vi "Module Top Level.vi"(8 "error in":errorcluster) -> (0 "error out":errorcluster)   [LabVIEW 2018, in "UDP Writer.lvlib"]
doc: "This is the top level VI for this module. It uses a queue for communications and is stopped user a user event. The general architecture is similar to a simple queued message handler.\n\nThe VIs associated with this module are organized in a LabVIEW Library."
uses:
  UDP Writer.lvlib
  Private Controls/Host Comms Data.ctl
  Top Level/Shared Controls/All Data Cluster.ctl
  Top Level/Shared Controls/Acq Data.ctl
  Private Controls/Module Data.ctl
  Private Controls/Module Action.ctl
panel:
  out "Connected?":bool
  # "UDP Writer"
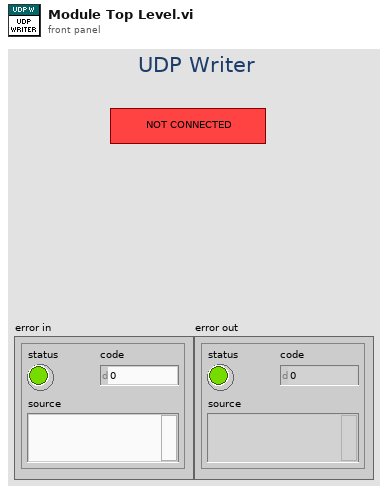
[diagram p1: front panel]
types:
  T1 = typedef "UDP Writer.lvlib/Host Comms Data.ctl" = cluster{"Connected?":bool, "connection ID":refnum<k16>, "PC IP":string, "PC Port":u16, "All Data Cluster":T2}
  T2 = typedef "All Data Cluster.ctl" = cluster{"AI":T3, "Accel Data":cluster{"Accel RMS(in/sec2)":dbl[], "Accel Peak(in/sec2)":dbl[], "Velocity RMS(in/sec)":dbl[], "Velocity Peak(in/sec)":dbl[]}, "Temps":cluster{"01-00-9213":dbl[], "01-01-9213":dbl[], "01-02-9213":dbl[]}, "00-03-9402(RPM)":dbl[], "02-04-9871":dbl[], "ARINC":sgl[]}
  T3 = typedef "Acq Data.ctl" = cluster{"00-00-9220":dbl[], "00-01-9220":dbl[], "02-02-9219":dbl[], "02-03-9227":dbl[], "02-05-9205":dbl[]}
  T4 = cluster{"z0":dbl, "dz":dbl, "plots":cluster{"x0":dbl, "dx":dbl, "Y":dbl[]}[]}
  T5 = cluster{"Accel RMS(in/sec2)":dbl[], "Accel Peak(in/sec2)":dbl[], "Velocity RMS(in/sec)":dbl[], "Velocity Peak(in/sec)":dbl[]}
  T6 = typedef "UDP Writer.lvlib/Module Data.ctl" = cluster{"Data":variant, "Action":T7}
  T7 = typedef "UDP Writer.lvlib/Module Action.ctl" = enum16{"Init", "Update ARINC", "Update Waterfall", "Update RPMs", "Update Temps", "Update Modbus", "Update AI", "Update Vibs", "Write", "Error"}
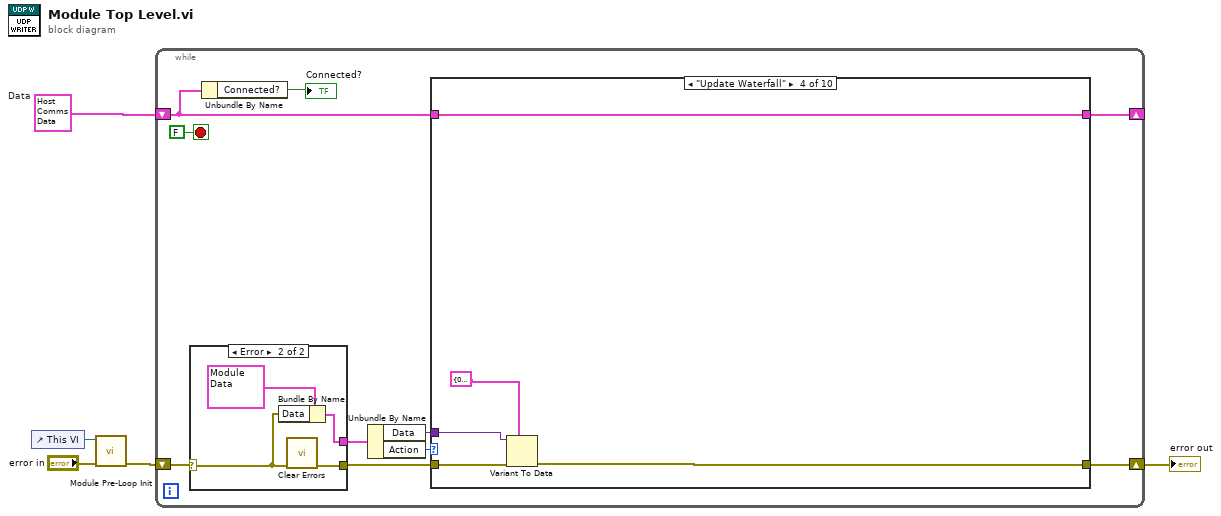
[diagram p0: block diagram]
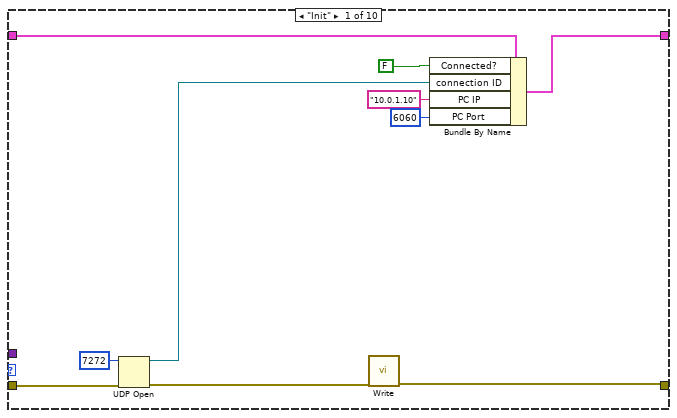
[diagram p2: hidden frame]
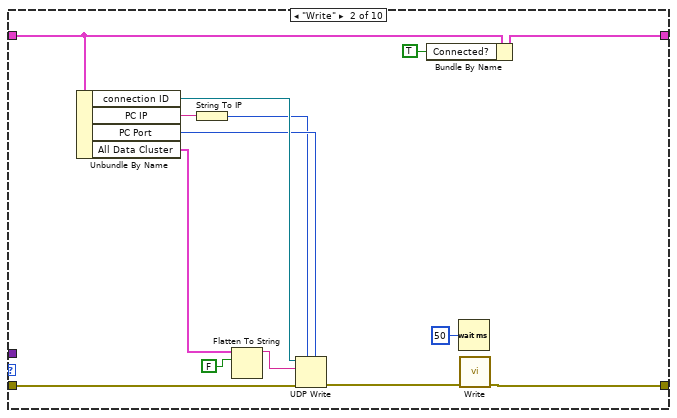
[diagram p3: hidden frame]
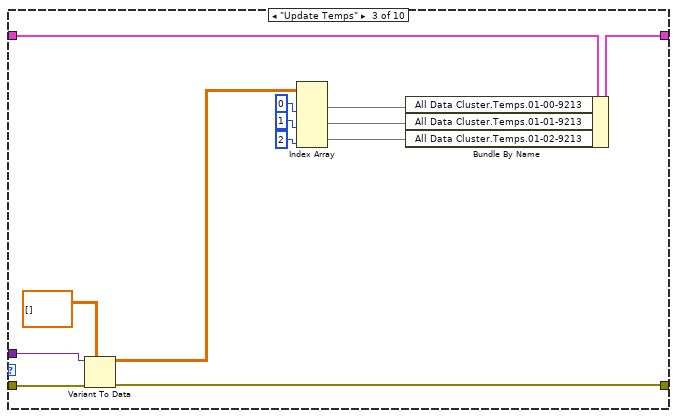
[diagram p4: hidden frame]
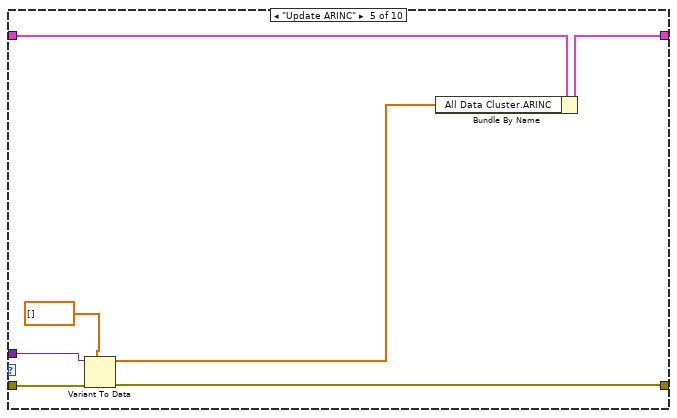
[diagram p5: hidden frame]
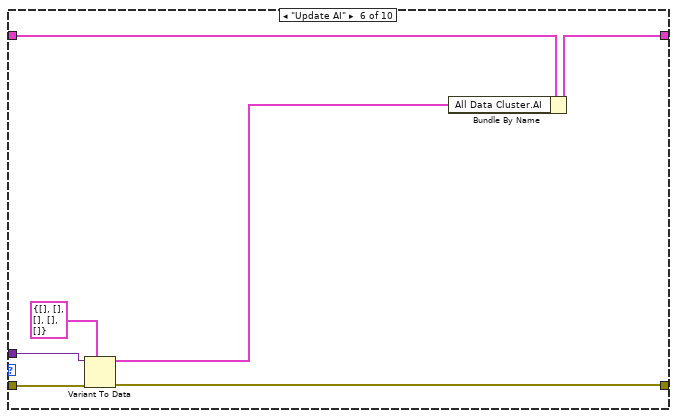
[diagram p6: hidden frame]
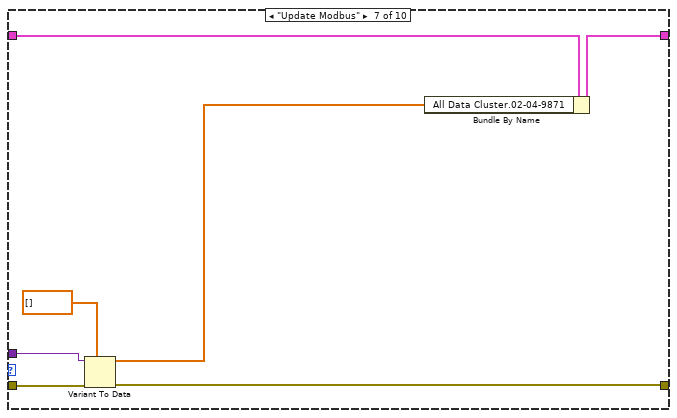
[diagram p7: hidden frame]
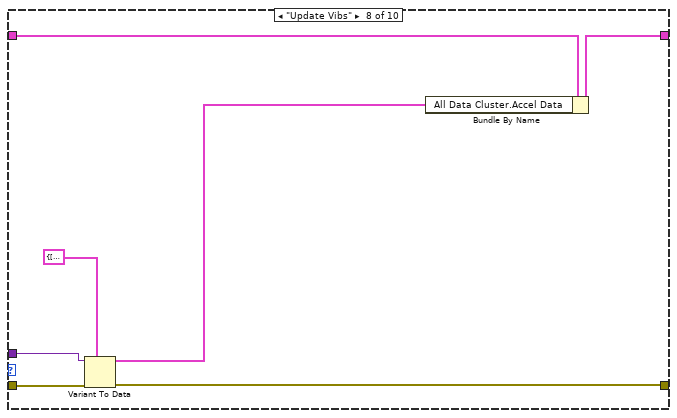
[diagram p8: hidden frame]
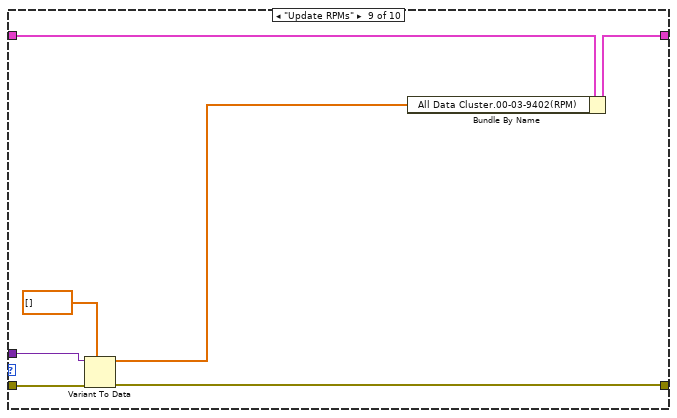
[diagram p9: hidden frame]
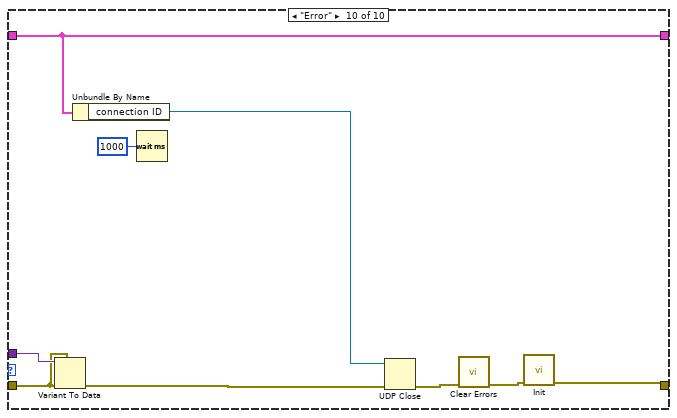
[diagram p10: hidden frame]
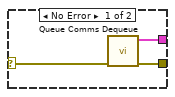
[diagram p11: hidden frame]
diagram:
  w2 = T1 {"Connected?"=FALSE, "connection ID"=refnum, "PC IP"="", "PC Port"=0, "All Data Cluster"={"AI"={"00-00-9220"=[], "00-01-9220"=[], "02-02-9219"=[], "02-03-9227"=[], "02-05-9205"=[]}, "Accel Data"={"Accel RMS(in/sec2)"=[], "Accel Peak(in/sec2)"=[], "Velocity RMS(in/sec)"=[], "Velocity Peak(in/sec)"=[]}, "Temps"={"01-00-9213"=[], "01-01-9213"=[], "01-02-9213"=[]}, "00-03-9402(RPM)"=[], "02-04-9871"=[], "ARINC"=[]}}  # Data
  n1 = control-ref of="This VI"() -> (w5:refnum<vi>)
  n2 = call "Module Pre-Loop Init.vi"("error in (no error)"="error in", "Top Level VI Ref in"=w5) -> ("error out"=w1:errorcluster)  [unwired: 9 in]
  n3 = while {
    shift-right: [w11] -> w3
    shift-left: w1 -> [w10]
    shift-right: [w9] -> _
    shift-left: w2 -> [w8]
    stop <- FALSE stop-if-true
    n4 = case shown="Error" w10 {
      selector: w10 -> [w103 w106]
      tunnel: [w104 w107] -> w15
      tunnel: [w102 w105] -> w12
      frame No Error {
        n5 = call "Queue Comms Dequeue.vi"("error in (no error)"=w103) -> ("error out"=w102:errorcluster, "element"=w104:T6)  [unwired: 9 in]
      }
      frame Error {
        n6 = Bundle By Name(cluster=T6 {"Data"=variant, "Action"=enum."Error"} ("element"), "Data"=w106) -> (w107:T6)
        n7 = call <vilib>:"Clear Errors.vi"("error in (no error)"=w106) -> ("error out"=w105:errorcluster)  [unwired: 5 in, 1 out]
      }
    }
    n8 = Unbundle By Name(w8) -> ("Connected?"=→"Connected?":bool)
    n9 = Unbundle By Name(w15) -> ("Data"=w13:variant, "Action"=w14:T7)
    n10 = case shown="\"Update Waterfall\"" w14 {
      tunnel: w13 -> [_ _ w50 w56 w62 w69 w76 w83 w90 w101]
      tunnel: w12 -> [w22 w38 w51 w57 w63 w70 w77 w84 w91 w100]
      tunnel: [w18 w30 w43 w53 w60 w67 w73 w81 w87 w99] -> w11
      tunnel: [w25 w33 w48 w54 w61 w68 w74 w82 w88 w97] -> w9
      tunnel: w8 -> [w24 w39 w52 w54 w64 w71 w78 w85 w92 w97]
      frame "Init" {
        n11 = UDP Open(8:w22, 11:u16 7272 ("port")) -> (port=w20:refnum<k16>, 0:w19:errorcluster)  [unwired: 3 in, 1 out]
        n12 = call "Write.vi"("error in"=w19) -> ("error out"=w18:errorcluster)  [unwired: 10 in]
        n13 = Bundle By Name(cluster=w24, "Connected?"=FALSE, "connection ID"=w20, "PC IP"="10.0.1.10", "PC Port"=u16 6060) -> (w25:T1)
      }
      frame "Write" {
        n14 = Unbundle By Name(w39) -> ("connection ID"=w37:refnum<k16>, "PC IP"=w35:string, "PC Port"=w36:u16, "All Data Cluster"=w28:T2)
        n15 = String To IP(1:w35) -> (0:w34:u32)
        n16 = Flatten To String(anything=w28, prepend array or string size? (T)=FALSE) -> (data string=w26:string)  [unwired: 2 in, 2 out]
        n17 = UDP Write(address=w34, port or service name=w36, connection ID=w37, data in=w26, 8:w38) -> (error out=w31:errorcluster)  [unwired: 1 in, 1 out]
        n18 = Bundle By Name(cluster=w39, "Connected?"=TRUE) -> (w33:T1)
        n19 = Wait (ms)(milliseconds to wait=u32 50) -> ()  [unwired: 1 out]
        n20 = call "Write.vi"("error in"=w31) -> ("error out"=w30:errorcluster)  [unwired: 10 in]
      }
      frame "Update Temps" {
        n21 = Variant To Data(error in=w51, type=dbl[][] [] ("appended array"), Variant=w50) -> (data=w47:dbl[][], error out=w43:errorcluster)
        n22 = Index Array(array=w47, index (col) #1=0 ("index (row)"), index (col) #2=1 ("index (row)"), index (col) #3=2 ("index (row)")) -> (element #1=w46:dbl[], element #2=w45:dbl[], element #3=w44:dbl[])  [unwired: 3 in]
        n23 = Bundle By Name(cluster=w52, "All Data Cluster.Temps.01-00-9213"=w46, "All Data Cluster.Temps.01-01-9213"=w45, "All Data Cluster.Temps.01-02-9213"=w44) -> (w48:T1)
      }
      frame "Update Waterfall" {
        n24 = Variant To Data(error in=w57, type=T4 {"z0"=0.0, "dz"=1.0, "plots"=[]} ("waterfall graph data out"), Variant=w56) -> (error out=w53:errorcluster)  [unwired: 1 out]
      }
      frame "Update ARINC" {
        n25 = Variant To Data(error in=w63, type=sgl[] [], Variant=w62) -> (data=w58:sgl[], error out=w60:errorcluster)
        n26 = Bundle By Name(cluster=w64, "All Data Cluster.ARINC"=w58) -> (w61:T1)
      }
      frame "Update AI" {
        n27 = Variant To Data(error in=w70, type=T3 {"00-00-9220"=[], "00-01-9220"=[], "02-02-9219"=[], "02-03-9227"=[], "02-05-9205"=[]} ("AI"), Variant=w69) -> (data=w65:T3, error out=w67:errorcluster)
        n28 = Bundle By Name(cluster=w71, "All Data Cluster.AI"=w65) -> (w68:T1)
      }
      frame "Update Modbus" {
        n29 = Variant To Data(error in=w77, type=dbl[] [] ("appended array"), Variant=w76) -> (data=w72:dbl[], error out=w73:errorcluster)
        n30 = Bundle By Name(cluster=w78, "All Data Cluster.02-04-9871"=w72) -> (w74:T1)
      }
      frame "Update Vibs" {
        n31 = Variant To Data(error in=w84, type=T5 {"Accel RMS(in/sec2)"=[], "Accel Peak(in/sec2)"=[], "Velocity RMS(in/sec)"=[], "Velocity Peak(in/sec)"=[]} ("All Data Cluster.Accel Data"), Variant=w83) -> (data=w80:T5, error out=w81:errorcluster)
        n32 = Bundle By Name(cluster=w85, "All Data Cluster.Accel Data"=w80) -> (w82:T1)
      }
      frame "Update RPMs" {
        n33 = Variant To Data(error in=w91, type=dbl[] [] ("appended array"), Variant=w90) -> (data=w86:dbl[], error out=w87:errorcluster)
        n34 = Bundle By Name(cluster=w92, "All Data Cluster.00-03-9402(RPM)"=w86) -> (w88:T1)
      }
      frame "Error" {
        n35 = Variant To Data(error in=w100, type=w100, Variant=w101) -> (error out=w98:errorcluster)  [unwired: 1 out]
        n36 = Unbundle By Name(w97) -> ("connection ID"=w96:refnum<k16>)
        n37 = Wait (ms)(milliseconds to wait=u32 1000) -> ()  [unwired: 1 out]
        n38 = UDP Close(connection ID=w96, 8:w98) -> (error out=w95:errorcluster)  [unwired: 1 out]
        n39 = call <vilib>:"Clear Errors.vi"("error in (no error)"=w95) -> ("error out"=w94:errorcluster)  [unwired: 5 in, 1 out]
        n40 = call "Init.vi"("error in"=w94) -> ("error out"=w99:errorcluster)  [unwired: 10 in]
      }
    }
  }
  "error out" <- w3
